vi "Stats Unbundle.vi"(8 "NAT Cluster in":T2, 9 "State":T4, 10 "Model":string, 11 "Auto Stats":T6) -> (0 "NAT Cluster out":T1, 1 "Cycle Time":dbl, 2 "Counters":cluster{"GoodCount":u32, "RejectCount":u32}, 3 "OEE Cluster":T3, 4 "Avg. Cycle Time":dbl, 5 "Total Times":T5, 7 "path":path)   [LabVIEW 2017]
uses:
  support/Controls/Auto Stats.ctl
  RT/Controls/Auto Times.ctl
  Controls/Logging FGV.ctl
  Controls/AVL Auto Time.ctl
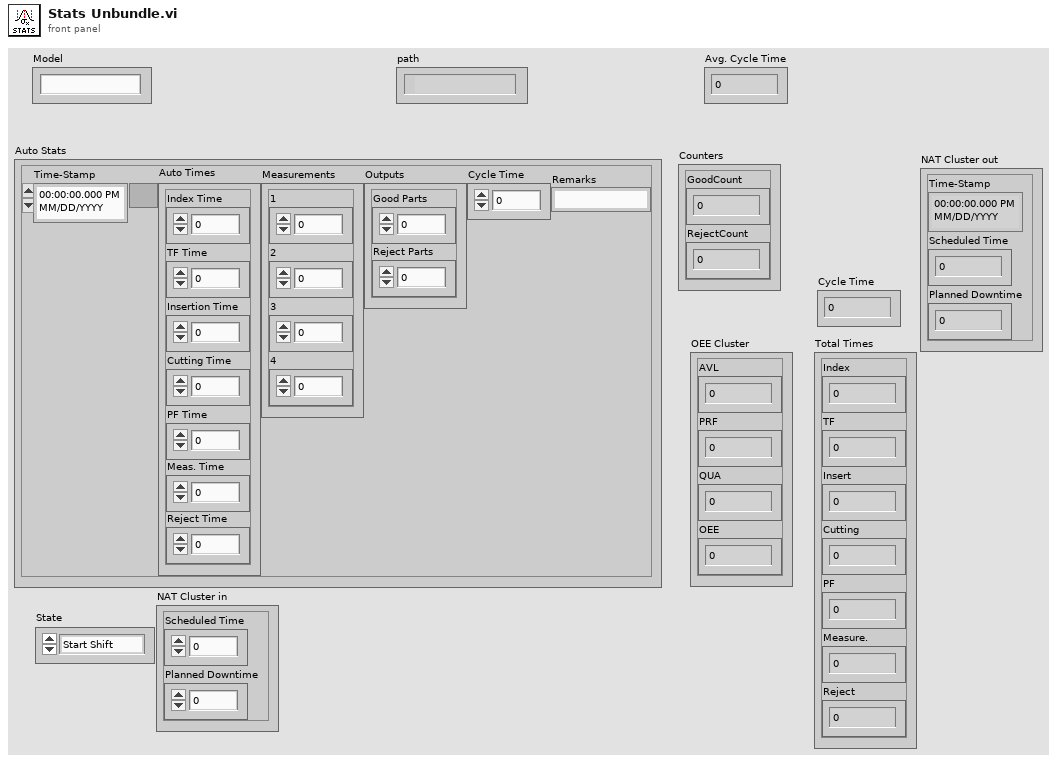
[diagram p1: front panel]
types:
  T1 = cluster{"Time-Stamp":timestamp, "Scheduled Time":dbl, "Planned Downtime":dbl}
  T2 = cluster{"Scheduled Time":dbl, "Planned Downtime":dbl}
  T3 = cluster{"AVL":dbl, "PRF":dbl, "QUA":dbl, "OEE":dbl}
  T4 = typedef "Logging FGV.ctl" = enum16{"Start Shift", "Log Index", "Read Shift", "Close Shift"}
  T5 = cluster{"Index":dbl, "TF":dbl, "Insert":dbl, "Cutting":dbl, "PF":dbl, "Measure.":dbl, "Reject":dbl}
  T6 = typedef "Auto Stats.ctl" = cluster{"Time-Stamp":timestamp, "Auto Times":T7, "Measurements":cluster{"1":dbl, "2":dbl, "3":dbl, "4":dbl}, "Outputs":cluster{"Good Parts":u32, "Reject Parts":u32}, "Cycle Time":dbl, "Remarks":string}
  T7 = typedef "Auto Times.ctl" = cluster{"Index Time":u32, "TF Time":u32, "Insertion Time":u32, "Cutting Time":u32, "PF Time":u32, "Meas. Time":u32, "Reject Time":u32}
  T8 = typedef "AVL Auto Time.ctl" = enum16{"Start Session", "Exited Auto", "Resumed Auto", "Read Time"}
  T9 = cluster{"[0]":dbl, "[1]":dbl, "[2]":dbl, "[3]":dbl, "[4]":dbl, "[5]":dbl, "[6]":dbl}
  T10 = cluster{"seconds since 1Jan1904":timestamp, dbl, dbl}
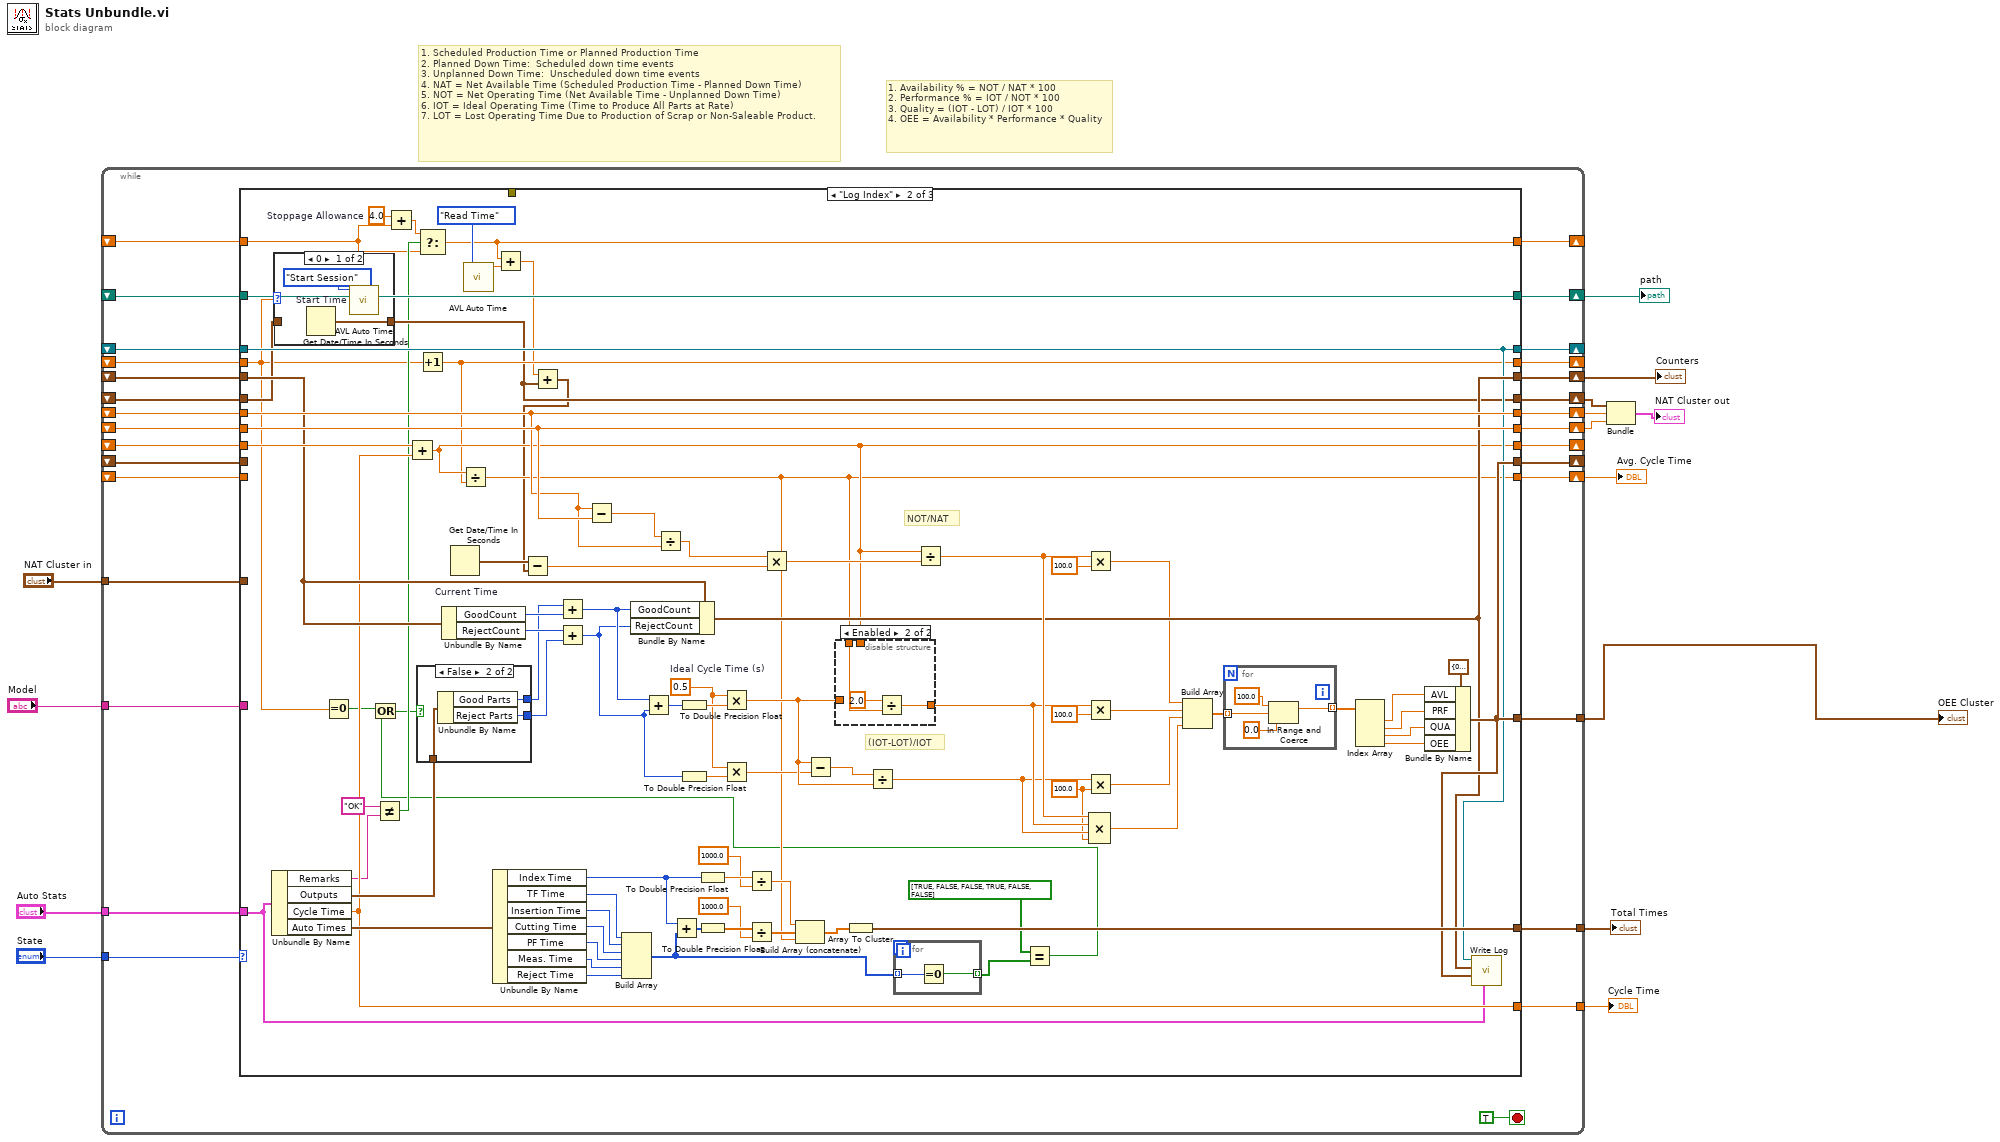
[diagram p0: block diagram]
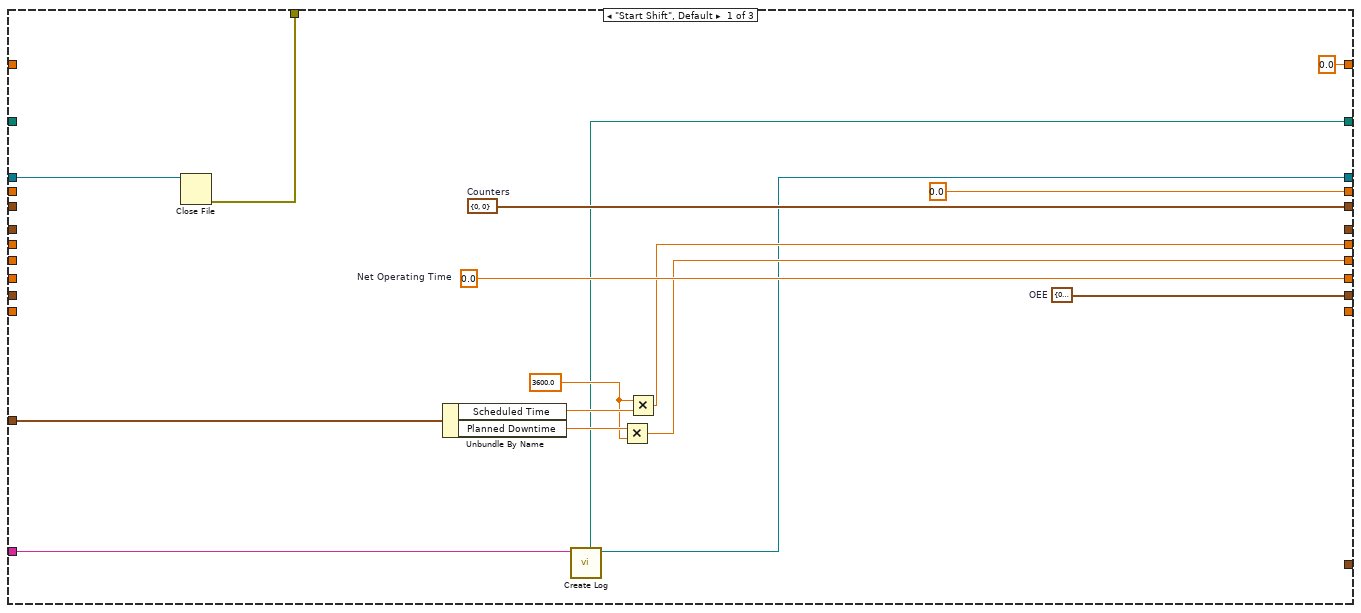
[diagram p2: hidden frame]
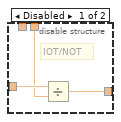
[diagram p3: hidden frame]
diagram:
  # "1.\tAvailability % = NOT / NAT * 100\n2.\tPerformance % = IOT / NOT * 100\n3.\tQuality = (IOT - LOT) / IOT * 100\n4.\tOEE = Availability * Performance * Quality"
  # "1.\tScheduled Production Time or Planned Production Time\n2.\tPlanned Down Time:  Scheduled down time events\n3.\tUnplanned Down Time:  Unscheduled down time events\n4.\tNAT = Net Available Time (Scheduled Production Time - Planned Down Time)\n5.\tNOT = Net Operating Time (Net Available Time - Unplanned Down Time)\n6.\tIOT = Ideal Operating Time (Time to Produce All Parts at Rate)\n7.\tLOT = Lost Operating Time Due to Production of Scrap or Non-Saleable Product."
  n1 = while {
    tunnel: "Auto Stats" -> [w44]
    tunnel: "State" -> [w43]
    shift-right: [w40] -> w8
    shift-left: _ -> [w37]
    shift-right: [w41] -> w9
    shift-left: _ -> [w38]
    shift-right: [w42] -> w6
    shift-left: _ -> [w39]
    shift-right: [w36] -> _
    shift-left: _ -> [w35]
    tunnel: [w34] -> w2
    shift-right: [w33] -> w13
    shift-left: _ -> [w32]
    tunnel: [w31] -> w12
    tunnel: [w29] -> w11
    shift-right: [w28] -> _
    shift-left: _ -> [w27]
    tunnel: "NAT Cluster in" -> [w26]
    shift-right: [w25] -> _
    shift-left: _ -> [w24]
    tunnel: "Model" -> [w23]
    shift-right: [w22] -> _
    shift-left: _ -> [w21]
    shift-right: [w20] -> w3
    shift-left: _ -> [w19]
    shift-right: [w18] -> w1
    shift-left: _ -> [w17]
    shift-right: [w16] -> _
    shift-left: _ -> [w15]
    stop <- TRUE stop-if-true
    n2 = case shown="\"Log Index\"" w43 {
      tunnel: w44 -> [_ w99 _]
      tunnel: [_ w78 w175] -> w42
      tunnel: [w53 w114 w172] -> w41
      tunnel: [w54 w129 w174] -> w40
      tunnel: w39 -> [_ w93 w175]
      tunnel: w38 -> [_ w114 w172]
      tunnel: w37 -> [_ w129 w174]
      tunnel: [w60 w95 w173] -> w36
      tunnel: w35 -> [_ w124 w173]
      tunnel: [_ w98 w170] -> w34
      tunnel: [w59 w97 w171] -> w33
      tunnel: w32 -> [_ w104 w171]
      tunnel: [_ w101 _] -> w31
      tunnel: [_ w100 _] -> w29
      tunnel: [w58 w98 w170] -> w28
      tunnel: w27 -> [_ _ w170]
      tunnel: w26 -> [w55 _ _]
      tunnel: [w51 w96 w169] -> w25
      tunnel: w24 -> [w50 w96 w169]
      tunnel: [w49 _ _] -> _
      tunnel: w23 -> [w48 _ _]
      tunnel: [0.0 w94 w168] -> w22
      tunnel: w21 -> [_ w64 w168]
      tunnel: [_ w79 w167] -> w20
      tunnel: w19 -> [_ _ w167]
      tunnel: [w46 w82 w166] -> w18
      tunnel: w17 -> [_ w82 w166]
      tunnel: [0.0 w69 w165] -> w16
      tunnel: w15 -> [_ w71 w165]
      frame "Start Shift", Default {
        w52 = 3600.0 ("y")
        w58 = T3 {"AVL"=0.0, "PRF"=0.0, "QUA"=0.0, "OEE"=0.0}  # OEE
        w59 = cluster{"GoodCount":u32, "RejectCount":u32} {"GoodCount"=0, "RejectCount"=0}  # Counters
        w60 = 0.0  # Net Operating Time
        n3 = Close File(refnum=w50) -> (error out=w49:errorcluster)  [unwired: 1 in, 1 out]
        n4 = Unbundle By Name(w55) -> ("Scheduled Time"=w57:dbl, "Planned Downtime"=w56:dbl)
        n5 = call "Create Log.vi"("Model"=w48) -> ("refnum out"=w51:refnum<file>, "path"=w46:path)  [unwired: 9 in]
        n6 = Multiply(x=w56, y=w52) -> (x*y=w54:dbl)
        n7 = Multiply(x=w52, y=w57) -> (x*y=w53:dbl)
      }
      frame "Log Index" {
        w74 = 4.0  # Stoppage Allowance
        w110 = 100.0 ("y")
        w115 = 0.5  # Ideal Cycle Time (s)
        # "NOT/NAT"
        # "(IOT-LOT)/IOT"
        n8 = Unbundle By Name(w99) -> ("Remarks"=w76:string, "Outputs"=w123:cluster{"Good Parts":u32, "Reject Parts":u32}, "Cycle Time"=w101:dbl, "Auto Times"=w146:T7)
        n9 = case shown="0" w64 {
          tunnel: w93 -> [_ w164]
          tunnel: [w163 w164] -> w78
          frame 0 {
            n10 = Get Date/Time In Seconds "Start Time"() -> (seconds since 1Jan1904=w163:timestamp)
            n11 = call "AVL Auto Time.vi"("State"=AVL_Auto_Time."Start Session") -> ()  [unwired: 10 in, 1 out]
          }
          frame Default {
          }
        }
        n12 = Equal To 0?(x=w64) -> (x = 0?=w63:bool)
        n13 = Not Equal?(x="OK", y=w76) -> (x != y?=w73:bool)
        n14 = Add(x=w74, y=w71) -> (x+y=w72:dbl)
        n15 = Add(x=w124, y=w101) -> (x+y=w95:dbl)
        n16 = Select(t=w72, s=w73, f=w71) -> (s? t:f=w69:dbl)
        n17 = Increment(x=w64) -> (x+1=w94:dbl)
        n18 = Unbundle By Name(w104) -> ("GoodCount"=w108:u32, "RejectCount"=w107:u32)
        n19 = Get Date/Time In Seconds "Current Time"() -> (seconds since 1Jan1904=w130:timestamp)
        n20 = Divide(x=w95, y=w94) -> (x/y=w79:dbl)
        n21 = call "AVL Auto Time.vi"("State"=AVL_Auto_Time."Read Time") -> ("Non-Auto Time"=w70:dbl)  [unwired: 10 in]
        n22 = Unbundle By Name(w146) -> ("Index Time"=w132:u32, "TF Time"=w140:u32, "Insertion Time"=w141:u32, "Cutting Time"=w142:u32, "PF Time"=w143:u32, "Meas. Time"=w144:u32, "Reject Time"=w145:u32)
        n23 = Add(x=w69, y=w70) -> (x+y=w68:dbl)
        n24 = Add(x=w68, y=w78) -> (x+y=w77:timestamp)
        n25 = Subtract(x=w130, y=w77) -> (x-y=w128:dbl)
        n26 = Subtract(x=w114, y=w129) -> (x-y=w127:dbl)
        n27 = Build Array(w140, w141, w142, w143, w144, w145) -> (w67:u32[])
        n28 = Divide(x=w127, y=w114) -> (x/y=w81:dbl)
        n29 = Add(x=w132, y=w67) -> (x+y=w137:u32[])
        n30 = To Double Precision Float(number=w132) -> (double precision float=w134:dbl)
        n31 = To Double Precision Float(number=w137) -> (double precision float=w139:dbl[])
        n32 = Divide(x=w134, y=1000.0) -> (x/y=w131:dbl)
        n33 = Divide(x=w139, y=1000.0) -> (x/y=w136:dbl[])
        n34 = Multiply(x=w81, y=w128) -> (x*y=w125:dbl)
        n35 = Build Array (concatenate)(w131, w136, w79) -> (w135:dbl[])
        n36 = Array To Cluster(array=w135) -> (cluster=w100:T9)
        n37 = for {
          tunnel: w67 -> [w148] mode=indexing
          tunnel: [w147] -> w66 mode=indexing
          n38 = Equal To 0?(x=w148) -> (x = 0?=w147:bool)
        }
        n39 = Divide(x=w95, y=w125) -> (x/y=w113:dbl)
        n40 = Equal?(x=bool[] [TRUE, FALSE, FALSE, TRUE, FALSE, FALSE], y=w66) -> (x = y?=w62:bool)
        n41 = Or(x=w63, y=w62) -> (x .or. y?=w61:bool)
        n42 = case shown="False" w61 {
          tunnel: w123 -> [_ w159]
          tunnel: [_ w161] -> w106
          tunnel: [_ w160] -> w105
          frame True {
          }
          frame False {
            n43 = Unbundle By Name(w159) -> ("Good Parts"=w161:u32, "Reject Parts"=w160:u32)
          }
        }
        n44 = Add(x=w106, y=w108) -> (x+y=w103:u32)
        n45 = Add(x=w107, y=w105) -> (x+y=w102:u32)
        n46 = Bundle By Name(cluster=w104, "GoodCount"=w103, "RejectCount"=w102) -> (w97:cluster{"GoodCount":u32, "RejectCount":u32})
        n47 = Add(x=w103, y=w102) -> (x+y=w122:u32)
        n48 = To Double Precision Float(number=w122) -> (double precision float=w121:dbl)
        n49 = To Double Precision Float(number=w102) -> (double precision float=w119:dbl)
        n50 = Multiply(x=w115, y=w121) -> (x*y=w117:dbl)
        n51 = Multiply(x=w115, y=w119) -> (x*y=w116:dbl)
        n52 = Subtract(x=w117, y=w116) -> (x-y=w118:dbl)
        n53 = disable-structure shown="Enabled" {
          disable-tunnel: w117 -> [w151 _]
          disable-tunnel: [w150 w152] -> w112
          disable-tunnel: w95 -> [w149 _]
          disable-tunnel: w79 -> [_ w154]
          frame Disabled {
            # "IOT/NOT"
            n54 = Divide(x=w151, y=w149) -> (x/y=w150:dbl)
          }
          frame Enabled {
            n55 = Divide(x=2.0 ("y"), y=w154) -> (x/y=w152:dbl)
          }
        }
        n56 = Divide(x=w118, y=w117) -> (x/y=w111:dbl)
        n57 = Multiply(x=w113, y=100.0) -> (x*y=w92:dbl)
        n58 = Multiply(x=w112, y=100.0) -> (x*y=w91:dbl)
        n59 = Multiply(x=w111, y=w110) -> (x*y=w90:dbl)
        n60 = Compound Arithmetic op=MULTIPLY(w113, w112, w111, w110) -> (w89:dbl)
        n61 = Build Array(w92, w91, w90, w89) -> (w88:dbl[])
        n62 = for {
          tunnel: w88 -> [w156] mode=indexing
          tunnel: [w155] -> w87 mode=indexing
          n63 = In Range and Coerce(upper limit=100.0, x=w156, lower limit=0.0) -> (coerced(x)=w155:dbl)  [unwired: 1 out]
        }
        n64 = Index Array(array=w87) -> (element #1=w86:dbl, element #2=w85:dbl, element #3=w84:dbl, element #4=w83:dbl)  [unwired: 4 in]
        n65 = Bundle By Name(cluster=T3 {"AVL"=0.0, "PRF"=0.0, "QUA"=0.0, "OEE"=0.0} ("OEE 2"), "AVL"=w86, "PRF"=w85, "QUA"=w84, "OEE"=w83) -> (w98:T3)
        n66 = call "Write Log.vi"("Auto Stats"=w99, "OEE in"=w98, "output cluster"=w97, "refnum out"=w96) -> ()  [unwired: 8 in]
      }
      frame "Read Shift" {
      }
    }
  }
  "OEE Cluster" <- w2
  "Counters" <- w13
  "Cycle Time" <- w12
  "Total Times" <- w11
  "Avg. Cycle Time" <- w3
  "path" <- w1
  n67 = Bundle("seconds since 1Jan1904"=w6, w9, w8) -> (→"NAT Cluster out":T10)  [unwired: 1 in]
